vi "Time_to_Website.vi"() -> ()   [LabVIEW 2022 SP3]
uses:
  <vilib>/Platform/browser.llb/Open URL in Default Browser (string).vi
panel:
  out "Time to open \nWebsite (ms)":i32
  in  "RUN":bool
  in  "URL":string
  # "Time_to_Website:\nJust enter a website's URL to see how long it takes to open.\nBe sure to include:\n-\"https://\"\n-Subdomain \"www.\"\n-Server Name ex \"google\"\n-Top Level Domain \".com\""
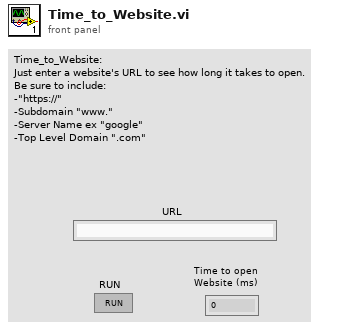
[diagram p1: front panel]
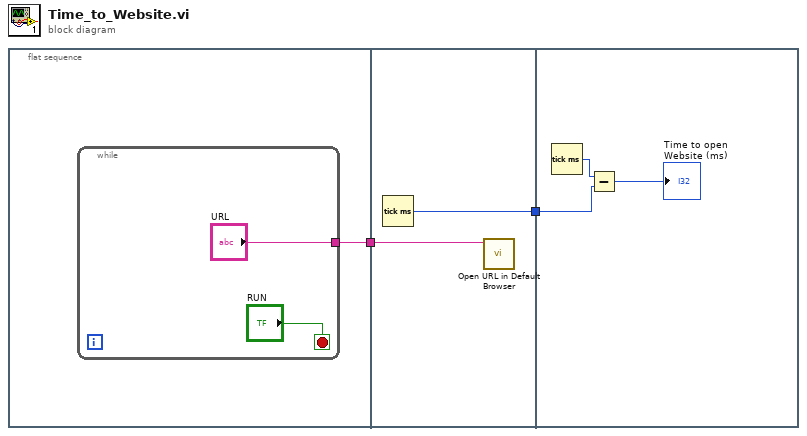
[diagram p0: block diagram]
diagram:
  n1 = flat-sequence {
    tunnel: [w3] -> w2
    tunnel: w2 -> [w6]
    tunnel: [w7] -> w1
    tunnel: w1 -> [w9]
    frame #0 {
      n2 = while {
        tunnel: ["URL"] -> w3
        stop <- "RUN" stop-if-true
      }
    }
    frame #1 {
      n3 = Tick Count (ms)() -> (millisecond timer value=w7:u32)
      n4 = call-poly <vilib>:"Open URL in Default Browser.vi"("URL"=w6) -> ()  [unwired: 5 in, 2 out]
    }
    frame #2 {
      n5 = Tick Count (ms)() -> (millisecond timer value=w10:u32)
      n6 = Subtract(x=w10, y=w9) -> (x-y=→"Time to open \nWebsite (ms)":u32)
    }
  }
